vi "Stop Core.vi"(10 "final error code":i32, 11 "StopEnabledActor in":refnum<class "StopEnabledActor.lvclass">) -> (3 "StopEnabledActor out":refnum<class "StopEnabledActor.lvclass">)   [LabVIEW 2017, in "StopEnabledActor.lvclass"]
doc: "(<B>Filename</B>: Actor Framework.lvlib:Actor.lvclass:Stop Core.vi)\n\nDefines what the actor does before it stops. Use the <B>final error code</B> input to determine whether the actor shut down in response to an error.\n\nBy default, this method does nothing. A descendant class may override it to define behavior, such as shutting down any processes the actor initiated in its override of the Actor Core method."
uses:
  StopEnabledActor.lvclass
  C:/Program Files (x86)/National Instruments/LabVIEW 2017/vi.lib/ActorFramework/Actor/Actor.lvclass
  <vilib>/ActorFramework/Actor/Actor.lvclass/Actor.ctl
  <vilib>/ActorFramework/Message Enqueuer/Message Enqueuer.lvclass/Message Enqueuer.ctl
  <vilib>/NI/Event Source Actor/Event Source/Event Source Messages/Unregister Msg/Unregister Msg.lvclass/Unregister Msg.ctl
  <vilib>/ActorFramework/Message Enqueuer/Init from Existing Queue.vi
  <vilib>/ActorFramework/Message Enqueuer/Enqueue.vi
  <vilib>/NI/Event Source Actor/Event Source/Event Source Messages/Unregister Msg/Unregister Msg.lvclass
  C:/Program Files (x86)/National Instruments/LabVIEW 2017/vi.lib/ActorFramework/Message/Message.lvclass
  <vilib>/ActorFramework/Message Priority Queue/Priority Enqueue.vi
  <vilib>/ActorFramework/Actor/Actor.lvclass
  <vilib>/ActorFramework/Message Enqueuer/Message Enqueuer.lvclass
  GlobalStopActor/GlobalStopActor.lvclass
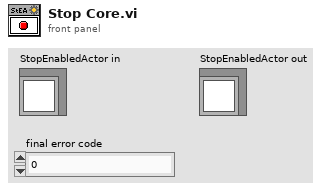
[diagram p1: front panel]
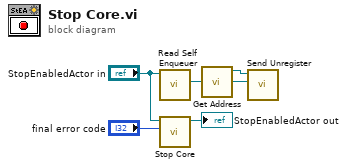
[diagram p0: block diagram]
diagram:
  n1 = call <vilib>:"Read Self Enqueuer.vi"("Actor"="StopEnabledActor in") -> ("Self Enqueuer"=w1:refnum<class "Message Enqueuer.lvclass">)  [unwired: 10 in]
  n2 = call-parent "Stop Core.vi"("final error code"="final error code", "Actor in"="StopEnabledActor in") -> ("Actor out"=→"StopEnabledActor out":refnum<class "StopEnabledActor.lvclass">)  [unwired: 9 in]
  n3 = call "Get Address.vi"() -> ("Enqueuer"=w3:refnum<class "Message Enqueuer.lvclass">)  [unwired: 11 in]
  n4 = call <vilib>:"Send Unregister.vi"("Registrant Address"=w1, "Event Source Address"=w3) -> ()  [unwired: 8 in, 2 out]
